vi "FTW-JSON-CompareEquality.vi"(0 "JSON Object":refnum<data-value>, 5 "JSON Object to Compare":refnum<data-value>, 11 "error in":errorcluster) -> (4 "JSON Object out":refnum<data-value>, 6 "Equal?":bool, 15 "error out":errorcluster)   [LabVIEW 2015]
uses:
  core/FTW-JSON-Core-Structure.ctl
panel:
  # "Inputs"
  # "Outputs"
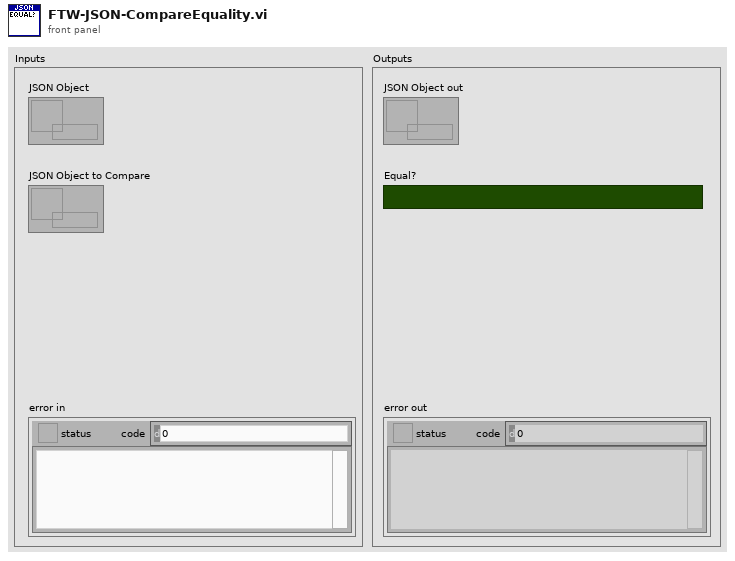
[diagram p1: front panel]
types:
  T1 = typedef "FTW-JSON-Core-Structure.ctl" = cluster{"JSON Object":i64, "Encoding Flags":i64, "Decoding Flags":i64}
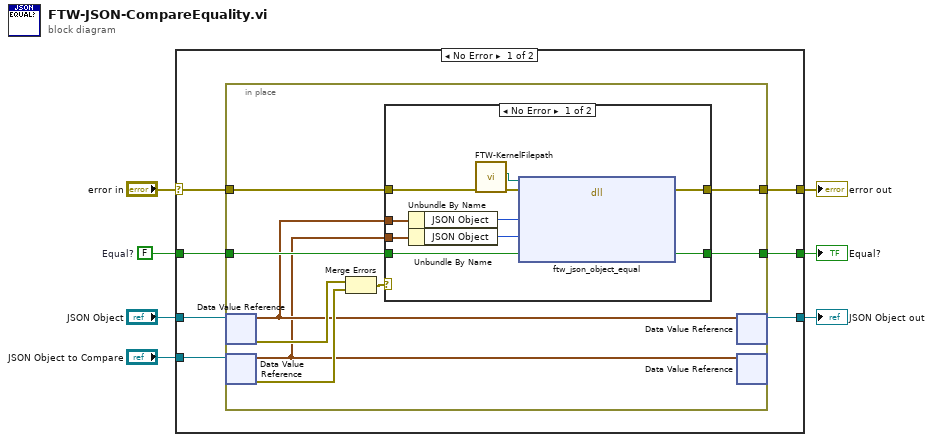
[diagram p0: block diagram]
diagram:
  w2 = FALSE  # Equal?
  n1 = case shown="No Error" "error in" {
    selector: "error in" -> [w14 w38]
    tunnel: [w13 w38] -> w7
    tunnel: "JSON Object" -> [w11 w36]
    tunnel: [w12 w37] -> w4
    tunnel: "JSON Object to Compare" -> [w10 _]
    tunnel: w2 -> [w9 w37]
    tunnel: [w8 w36] -> w1
    frame No Error {
      n2 = in-place {
        in-place-border: w14 -> [w23]
        in-place-border: [w22] -> w13
        in-place-border: [w21] -> w12
        in-place-border: w9 -> [w17]
        n3 = in-place-dvr #1(w11) -> (w16:T1, w20:errorcluster)
        n4 = in-place-dvr #2(w10) -> (w15:T1, w19:errorcluster)
        n5 = Merge Errors(w20, w19) -> (w18:errorcluster)
        n6 = case shown="No Error" w18 {
          tunnel: w23 -> [w25 w35]
          tunnel: [w33 w35] -> w22
          tunnel: [w27 w34] -> w21
          tunnel: w17 -> [w28 w34]
          tunnel: w16 -> [w30 _]
          tunnel: w15 -> [w29 _]
          frame No Error {
            n7 = Unbundle By Name(w30) -> ("JSON Object"=w32:i64)
            n8 = Unbundle By Name(w29) -> ("JSON Object"=w31:i64)
            n9 = call "FTW-KernelFilepath.vi"("error in"=w25) -> ("error out"=w24:errorcluster, "Library Filepath"=w26:path)  [unwired: 8 in, 1 out]
            n10 = dll-call lib="?" fn="ftw_json_object_equal"(path in=w26, error in=w24, "JSON Object Pointer 1"=w32, "JSON Object Pointer 2"=w31, "Are Objects Equal?"=w28) -> (error out=w33:errorcluster, "Are Objects Equal?"=w27:bool)  [unwired: 4 in, 1 out]
          }
          frame Error {
          }
        }
        n11 = in-place-dvr #1(w16) -> (w8:refnum<data-value>)  [unwired: 1 out]
        n12 = in-place-dvr #2(w15) -> ()  [unwired: 2 out]
      }
    }
    frame Error {
    }
  }
  "error out" <- w7
  "Equal?" <- w4
  "JSON Object out" <- w1
